vi "simple update step.vi"(1 "apply measurement?":bool=TRUE, 5 "location":i16, 7 "state in":T1, 9 "num photons":u16) -> (8 "state out":T1)   [LabVIEW 2010]
uses:
  kalman simple pv state.ctl
  <vilib>/rvi/FXPMathLib/FxpSub/XNode/nifxpmath_Sub.xnode
  <vilib>/rvi/FXPMathLib/FxpSub/subVIs/nifxpmath_Sub_SimConfig.ctl
  <vilib>/fxp/LVFixedPointQuantizationPolicyTypeDef.ctl
  <vilib>/fxp/LVFixedPointOverflowPolicyTypeDef.ctl
  <vilib>/rvi/FXPMathLib/FxpMul/XNode/nifxpmath_Multiplier.xnode
  <vilib>/rvi/FXPMathLib/FxpMul/subVIs/nifxpmath_Mul_SimConfig.ctl
  <vilib>/rvi/FXPMathLib/FxpAdd/XNode/nifxpmath_Add.xnode
  <vilib>/rvi/FXPMathLib/FxpAdd/subVIs/nifxpmath_Add_SimConfig.ctl
  <vilib>/rvi/FXPMathLib/FxpSub/simVIs/DllFxpSubTemp_sub.vi
  <vilib>/rvi/FXPMathLib/FxpMul/simVIs/DllFxpMulTemp_sub.vi
  <vilib>/rvi/FXPMathLib/FxpAdd/simVIs/DllFxpAddTemp_sub.vi
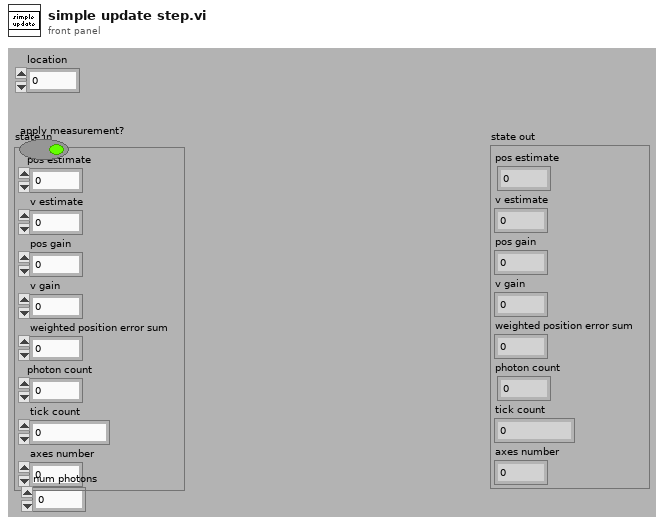
[diagram p1: front panel]
types:
  T1 = typedef "kalman simple pv state.ctl" = cluster{"pos estimate":fxp<+/-,32,16>, "v estimate":fxp<+/-,32,-4>, "pos gain":fxp<+,32,0>, "v gain":fxp<+,32,0>, "weighted position error sum":fxp<+/-,32,32>, "photon count":u32, "tick count":u32, "axes number":u8}
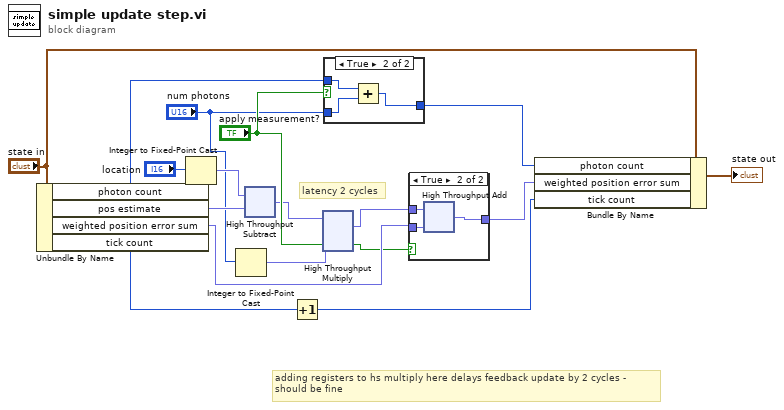
[diagram p0: block diagram]
diagram:
  # "latency 2 cycles"
  # "adding registers to hs multiply here delays feedback update by 2 cycles - \nshould be fine"
  n1 = Unbundle By Name("state in") -> ("photon count"=w8:u32, "pos estimate"=w13:fxp<+/-,32,16>, "weighted position error sum"=w12:fxp<+/-,32,32>, "tick count"=w2:u32)
  n2 = Integer to Fixed-Point Cast(integer="location") -> (fixed-point=w14:fxp<+/-,16,16>)  [unwired: 1 in]
  n3 = Integer to Fixed-Point Cast(integer="num photons") -> (fixed-point=w4:fxp<+,16,16>)  [unwired: 1 in]
  n4 = xnode "High Throughput Subtract"("x"=w14, "y"=w13) -> ("x-y"=w9:fxp<+/-,32,16>)
  n5 = Increment(x=w2) -> (x+1=w1:u32)
  n6 = xnode "High Throughput Multiply"("x"=w9, "y"=w4, "input valid"="apply measurement?") -> ("x*y"=w3:fxp<+/-,32,32>, "output valid"=w6:bool)  [unwired: 1 in, 1 out]
  n7 = case shown="True" "apply measurement?" {
    tunnel: w8 -> [w18 w21]
    tunnel: [w18 w19] -> w7
    tunnel: "num photons" -> [_ w20]
    frame False {
    }
    frame True {
      n8 = Add(x=w21, y=w20) -> (x+y=w19:u32)
    }
  }
  n9 = case shown="True" w6 {
    tunnel: w12 -> [w22 w25]
    tunnel: [w22 w24] -> w11
    tunnel: w3 -> [_ w23]
    frame False {
    }
    frame True {
      n10 = xnode "High Throughput Add"("x"=w23, "y"=w25) -> ("x+y"=w24:fxp<+/-,32,32>)
    }
  }
  n11 = Bundle By Name(cluster="state in", "photon count"=w7, "weighted position error sum"=w11, "tick count"=w1) -> (→"state out":T1)
